vi "LECTURA&ESCRITURA_ARDUINO.vi"() -> ()   [LabVIEW 2021]
uses:
  <vilib>/Instr/_visa.llb/VISA Configure Serial Port (Instr).vi
panel:
  out "PIN 3 PWM":i32
  in  "stop":bool
  out "A0":i32
  out "Waveform Chart":dynamicdata(graph)
  in  "STEP":dbl(slide) scale=0.0..100.0
  in  "PUERTO COM \nEN ARDUINO":refnum<visa-resource-name>
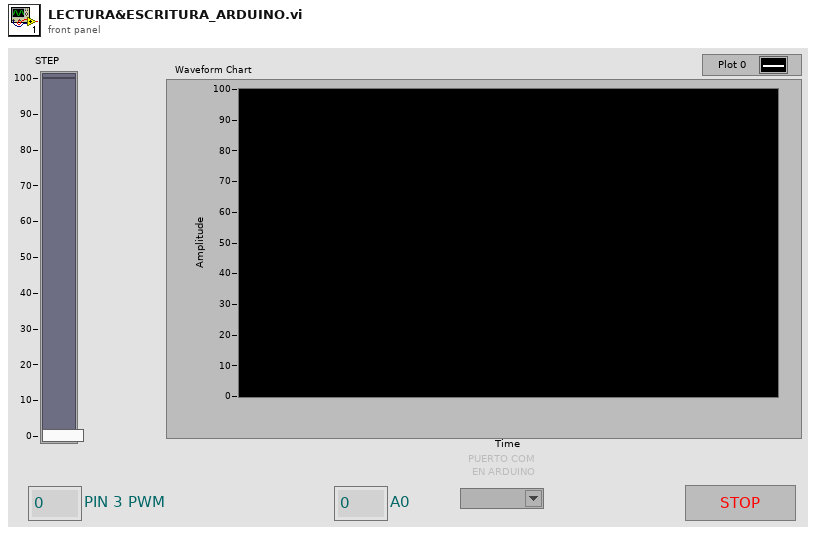
[diagram p1: front panel]
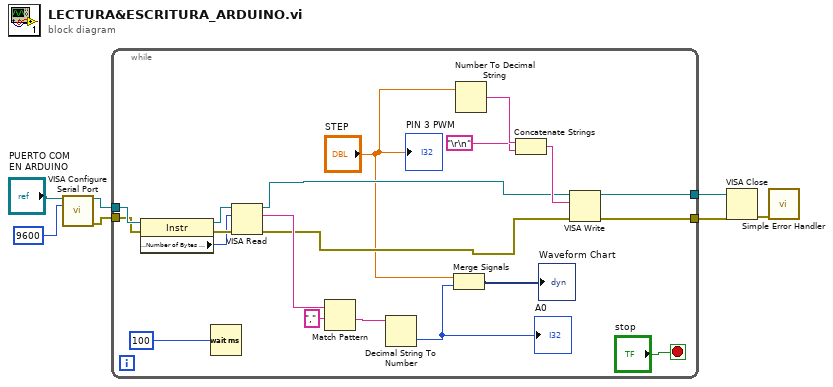
[diagram p0: block diagram]
diagram:
  n1 = call-poly "VISA Configure Serial Port"("VISA resource name"="PUERTO COM \nEN ARDUINO", "baud rate (9600)"=u32 9600) -> ("VISA resource name out"=w4:refnum<visa-resource-name>, "error out"=w3:errorcluster)  [unwired: 12 in]
  n2 = while {
    tunnel: w4 -> [w14]
    tunnel: w3 -> [w13]
    tunnel: [w12] -> w2
    tunnel: [w11] -> w1
    stop <- "stop" stop-if-true
    n3 = property class="Instr"(reference=w14, error in=w13) -> (reference out=w26:refnum<visa-resource-name>, error out=w25:errorcluster, "Serial Settings:Number of Bytes at Serial Port"=w24:u32)
    n4 = Wait (ms)(milliseconds to wait=u32 100) -> ()  [unwired: 1 out]
    n5 = VISA Read(VISA resource name=w26, byte count=w24, error in (no error)=w25) -> (VISA resource name out=w17:refnum<visa-resource-name>, read buffer=w23:string, error out=w16:errorcluster)  [unwired: 1 out]
    n6 = Match Pattern(string=w23, regular expression=",") -> (after substring=w21:string)  [unwired: 1 in, 3 out]
    n7 = Decimal String To Number(string=w21) -> (number=w9:i32)  [unwired: 2 in, 1 out]
    "A0" <- w9
    n8 = Merge Signals("STEP", w9) -> (→"Waveform Chart":dynamicdata)
    n9 = Number To Decimal String(number="STEP") -> (decimal integer string=w19:string)  [unwired: 1 in]
    n10 = Concatenate Strings(w19, "\r\n") -> (w20:string)
    n11 = VISA Write(VISA resource name=w17, write buffer=w20, error in (no error)=w16) -> (VISA resource name out=w12:refnum<visa-resource-name>, error out=w11:errorcluster)  [unwired: 1 out]
    "PIN 3 PWM" <- "STEP"
  }
  n12 = VISA Close(VISA resource name=w2, error in (no error)=w1) -> (error out=w6:errorcluster)
  n13 = call <vilib>:"Simple Error Handler.vi"("error in (no error)"=w6) -> ()  [unwired: 4 in, 5 out]
